vi "SVX Polar Plot (N Ch - M Orders).vi"(0 "magnitudes [RMS]":T9(array[cluster]) {"magnitude" format="%.2f"; "time/rev/RPM" format="%.2f"}, 5 "phases [phase lag]":cluster{"time/rev/RPM":dbl[], "phase":dbl[]}[][](array[cluster]) {"phase" format="%.2f"; "time/rev/RPM" format="%.2f"}, 9 "magnitude info":T2[](array[typedef]) {"x-axis units" items=["Time (s)"=0, "Frequency-CB (Hz)"=1, "Frequency-CPB (Hz)"=1248, "Frequency-Arbitrary (Hz)"=2357, "Quefrency (s)"=2, "Revolutions (rev)"=3, "Order"=4, "Speed (RPM)"=11, "Speed (rad/s)"=21, "Index"=65535]; "weighting filter" items=["Linear", "A-weighting", "B-weighting", "C-weighting", "ITU-R 468-4", "Dolby", "CCITT", "C-message", "Wb", "Wc", "Wd", "We", "Wf", "Wh", "Wj", "Wk", "Wm", "AES17 20 kHz lowpass", "AES17 40 kHz lowpass", "AES17 20 kHz highpass", "AES17 40 kHz highpass"]; "dB reference [EU]" format="%.2f"; "engineering units" items=["custom..."=0, "V"=1, "A"=21, "C"=30, "pC"=31, "s"=32, "-"=29, "Pa"=2, "N"=20, "g"=3, "m/s^2"=4, "m/s"=5, "m"=6, "mm/s"=12, "mm"=13, "micron/s"=14, "micron"=15, "in/s^2"=7, "in/s"=8, "in"=9, "mil/s"=10, "mil"=11, "rad/s^2"=16, "rad/s"=17, "rad"=18, "deg/s^2"=26, "deg/s"=27, "deg"=28, "RPM"=22, "cycle/s^2"=23, "Hz"=24, "cycle"=25, "strain"=19]; "spectral info"."window" items=["None "=0, "Hanning"=1, "Hamming"=2, "Blackman-Harris"=3, "Exact Blackman"=4, "Blackman"=5, "Flat Top"=6, "4 Term B-Harris "=7, "7 Term B-Harris"=8, "Low Sidelobe"=9, "Force - Exponential"=10, "Gaussian"=62]}, 11 "error in (no error)":errorcluster, 12 "channel properties":T1[](array[typedef]) {"probe angle [deg]" max=360; "direction" items=["CCW", "CW"]}) -> (3 "unit labels":string[](array[string]), 4 "polar plot":T8(array[cluster]), 15 "error out":errorcluster)   [LabVIEW 2017, in "SoundVib_OAVisualization.lvlib"]
doc: "Prepares polar plot data for displaying on a Polar Plot. Use this VI to show magnitude versus phase for a specific order. Wire data to the <B>magnitudes [RMS]</B> and <B>phases [phase lag]</B> inputs to determine the polymorphic instance to use or manually select the instance."
uses:
  <vilib>/addons/Sound and Vibration/Order Analysis/Data Presentation/SoundVib_OAVisualization.lvlib
  <vilib>/addons/_NISVFA/_Shared subVIs/Controls/svc_Spectrum Info.ctl
  <vilib>/addons/_NISVFA/_Shared subVIs/Controls/svc_X-Axis Units.ctl
  <vilib>/addons/_NISVFA/_Shared subVIs/Controls/svc_Spectrum Type.ctl
  <vilib>/addons/_NISVFA/_Shared subVIs/Controls/svc_Engineering Units Text Ring.ctl
  <vilib>/addons/_NISVFA/_Shared subVIs/Controls/svc_Weighting Filter Text Ring.ctl
  <vilib>/addons/_NISVFA/_Shared subVIs/Controls/svc_Complimentary Spectrum Units.ctl
  <vilib>/addons/Sound and Vibration/Order Analysis/Data Presentation/SubVIs/OAT MCM Channel Property.ctl
  <vilib>/addons/_NISVFA/_Spectrum Processing/SVFA Unit Conversion (XY) (N Ch - M Orders).vi
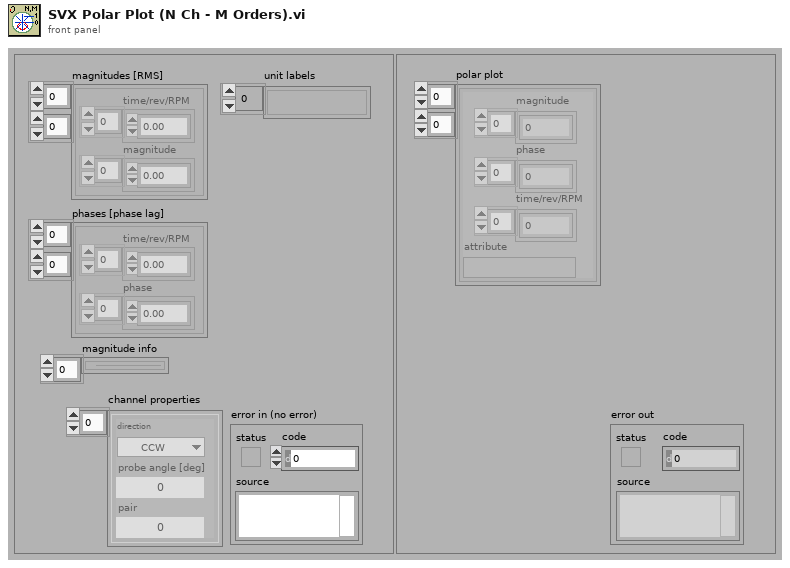
[diagram p1: front panel]
types:
  T1 = typedef "OAT MCM Channel Property.ctl" = cluster{"direction":u16, "probe angle [deg]":u16, "pair":u16}
  T2 = typedef "svc_Spectrum Info.ctl" = cluster{"channel name":string, "description":string, "x-axis units":T3, "spectral info":cluster{"spectrum type":T4, "linear/dB":enum16{"linear", "dB"}, "window":u16, "window size":i32, "FFT size":i32}, "engineering units":T5, "custom label":string, "dB reference [EU]":dbl, "peak units":enum16{"rms", "peak", "peak-peak"}, "weighting filter":T6, "spectral density?":bool, "unit label":string, "spectrum skewed?":bool, "complimentary spectrum units":T7}
  T3 = typedef "svc_X-Axis Units.ctl" = u16
  T4 = typedef "svc_Spectrum Type.ctl" = enum16{"FFT Spectrum [complex]", "Amplitude [Magnitude]", "Power [Magnitude^2]", "Cross Spectrum [complex]", "Frequency Response [Complex]"}
  T5 = typedef "svc_Engineering Units Text Ring.ctl" = u16
  T6 = typedef "svc_Weighting Filter Text Ring.ctl" = u16
  T7 = typedef "svc_Complimentary Spectrum Units.ctl" = enum16{"none", "radians", "degrees", "cycles", "imaginary"}
  T8 = cluster{"magnitude":dbl[], "phase":dbl[], "time/rev/RPM":dbl[], "attribute":variant}[][]
  T9 = cluster{"time/rev/RPM":dbl[], "magnitude":dbl[]}[][]
  T10 = cluster{"linear/dB":enum16{"no change", "linear", "dB"}, "dB reference (0: no change)":dbl, "power/magnitude":enum16{"no change", "power", "magnitude"}, "view":enum16{"no change", "rms", "peak", "peak-peak"}}
  T11 = cluster{"magnitude":dbl[], "phase":dbl[], "time/rev/RPM":dbl[], "attribute":variant}
  T12 = cluster{"time/rev/rpm":dbl[], "magnitude":dbl[]}[][]
  T13 = cluster{"dB on? (F)":bool, "unwrap phase? (T)":bool, "unit in degree? (T)":bool}
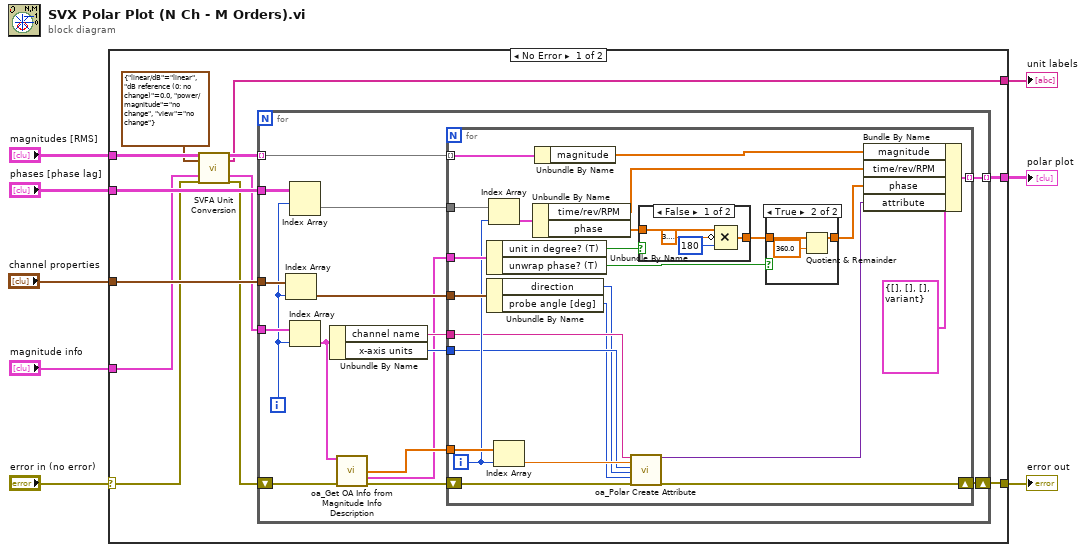
[diagram p0: block diagram]
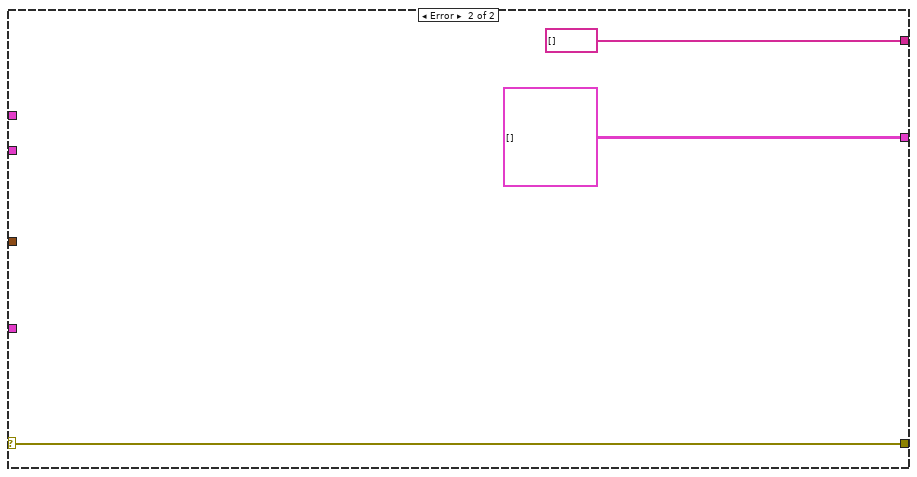
[diagram p4: hidden frame]
diagram:
  n1 = case shown="No Error" "error in (no error)" {
    selector: "error in (no error)" -> [w15 w72]
    tunnel: "magnitudes [RMS]" -> [w16 _]
    tunnel: "phases [phase lag]" -> [w20 _]
    tunnel: "channel properties" -> [w19 _]
    tunnel: [w18 w72] -> w5
    tunnel: [w17 T8 []] -> w3
    tunnel: "magnitude info" -> [w12 _]
    tunnel: [w9 string[] [] ("unit labels")] -> w1
    frame No Error {
      n2 = call-poly <vilib>:"SVFA Unit Conversion.vi"("magnitudes"=w16, "desired scaling"=T10 {"linear/dB"=enum."linear", "dB reference (0: no change)"=0.0, "power/magnitude"=enum."no change", "view"=enum."no change"}, "magnitudes info in"=w12, "error in (no error)"=w15) -> ("converted magnitudes"=w13:T12, "unit labels"=w9:string[], "magnitudes info out"=w11:T2[], "error out"=w14:errorcluster)  [unwired: 12 in]
      n3 = for {
        tunnel: w13 -> [w36] mode=indexing
        tunnel: w20 -> [w32]
        tunnel: w19 -> [w29]
        tunnel: w11 -> [w30]
        shift-right: [w35] -> w18
        shift-left: w14 -> [w25]
        tunnel: [w33] -> w17 mode=indexing
        i -> [w28]
        n4 = Index Array(array=w29, index=w28) -> (element=w27:T1)
        n5 = Index Array(array=w32, index (row)=w28) -> (element=w31:cluster{"time/rev/RPM":dbl[], "phase":dbl[]}[])  [unwired: 1 in]
        n6 = Index Array(array=w30, index=w28) -> (element=w23:T2)
        n7 = Unbundle By Name(w23) -> ("channel name"=w34:string, "x-axis units"=w26:T3)
        n8 = call <vilib>:"oa_Get OA Info from Magnitude Info Description.vi"("magnitude info"=w23, "error in (no error)"=w25) -> ("orders to compute"=w22:dbl[], "view"=w21:T13, "error out"=w24:errorcluster)  [unwired: 9 in, 2 out]
        n9 = for {
          tunnel: w36 -> [w60] mode=indexing
          tunnel: w31 -> [w54]
          tunnel: w27 -> [w59]
          tunnel: w21 -> [w58]
          tunnel: [w55] -> w33 mode=indexing
          shift-right: [w46] -> w35
          shift-left: w24 -> [w47]
          tunnel: w34 -> [w44]
          tunnel: w22 -> [w52]
          tunnel: w26 -> [w43]
          i -> [w51]
          n10 = Unbundle By Name(w58) -> ("unit in degree? (T)"=w57:bool, "unwrap phase? (T)"=w39:bool)
          n11 = Unbundle By Name(w59) -> ("direction"=w41:u16, "probe angle [deg]"=w42:u16)
          n12 = Index Array(array=w54, index=w51) -> (element=w53:cluster{"time/rev/RPM":dbl[], "phase":dbl[]})
          n13 = Index Array(array=w52, index=w51) -> (element=w45:dbl)
          n14 = Unbundle By Name(w53) -> ("time/rev/RPM"=w48:dbl[], "phase"=w49:dbl[])
          n15 = Unbundle By Name(w60) -> ("magnitude"=w50:dbl[])
          n16 = call <vilib>:"oa_Polar Create Attribute.vi"("channel name"=w44, "order"=w45, "x-axis units"=w43, "rotation direction"=w41, "probe angle [deg]"=w42, "error in (no error)"=w47) -> ("attribute out"=w40:variant, "error out"=w46:errorcluster)  [unwired: 12 in]
          n17 = case shown="False" w57 {
            tunnel: w49 -> [w68 w69]
            tunnel: [w65 w69] -> w38
            frame False {
              n18 = Compound Arithmetic op=MULTIPLY(w68, invert 3.141592653589793, 180) -> (w65:dbl[])
            }
            frame True {
            }
          }
          n19 = case shown="True" w39 {
            tunnel: w38 -> [w61 w63]
            tunnel: [w61 w62] -> w37
            frame False {
            }
            frame True {
              n20 = Quotient & Remainder(x=w63, y=360.0) -> (x-y*floor(x/y)=w62:dbl[])  [unwired: 1 out]
            }
          }
          n21 = Bundle By Name(cluster=T11 {"magnitude"=[], "phase"=[], "time/rev/RPM"=[], "attribute"=variant} ("element"), "magnitude"=w50, "time/rev/RPM"=w48, "phase"=w37, "attribute"=w40) -> (w55:T11)
        }
      }
    }
    frame Error {
    }
  }
  "polar plot" <- w3
  "error out" <- w5
  "unit labels" <- w1
